vi "SmartLibrary.vi"() -> ()   [LabVIEW 2020]
uses:
  Control 1.ctl
  <vilib>/Utility/file.llb/Read Delimited Spreadsheet (string).vi
panel:
  in  "?":T1(tab)
  out "Misplaced":u8(slide) scale=0.0..100.0
  in  "ENTER BOOK TITLE":string
  out "Current Date and Time":timestamp format="%<%X\n%x>T"
  in  "Search Button":bool
  out "Available":u8(slide) scale=0.0..100.0
  out "Borrowed":u8(slide) scale=0.0..100.0
  in  "RFID 1":bool
  in  "RFID 2":bool
  in  "RFID 3":bool
  in  "RFID 4":bool
  in  "RFID 5":bool
  in  "RFID 6":bool
  in  "RFID 7":bool
  in  "RFID 8":bool
  out "ONLINE":bool
  out "OFFLINE":bool
  out "Author:":string
  out "Call mumber:":string
  out "ISBN/ISSN:":string
  in  "Select\nCSV Database":T2 caption="file path (dialog if empty)"
  # "Book Inventory %"
  # "BOOKS"
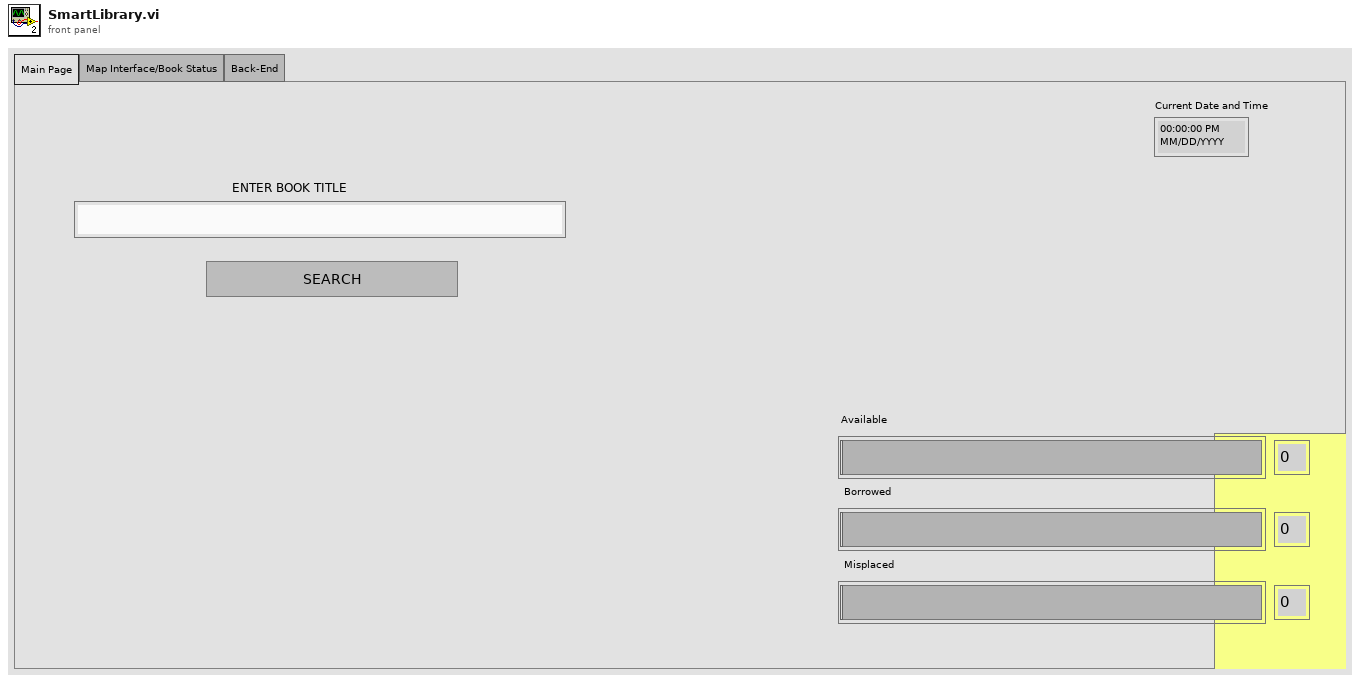
[diagram p1: front panel]
types:
  T1 = enum32{"Main Page", "Map Interface/Book Status", "Back-End"}
  T2 = typedef "Control 1.ctl" = path
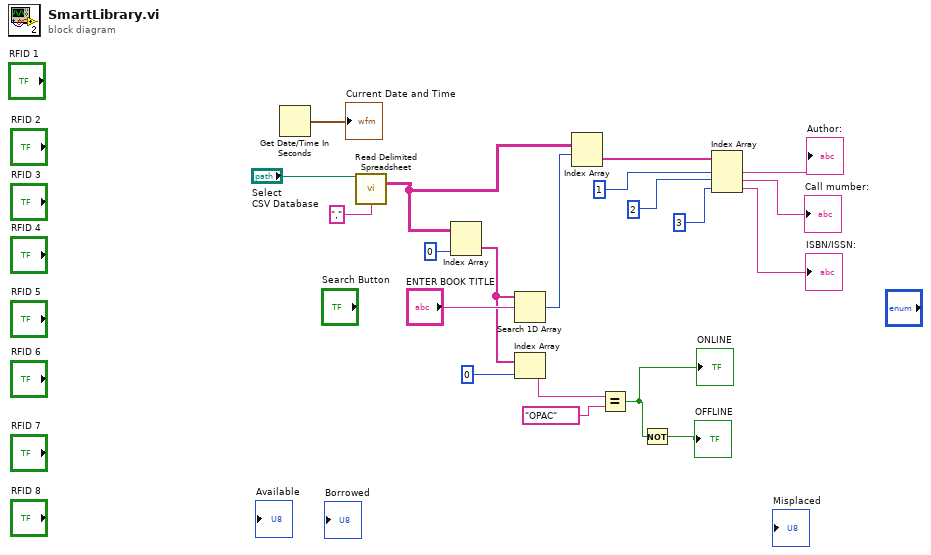
[diagram p0: block diagram]
diagram:
  n1 = Get Date/Time In Seconds() -> (seconds since 1Jan1904=→"Current Date and Time":timestamp)
  n2 = call-poly <vilib>:"Read Delimited Spreadsheet.vi"("file path (dialog if empty)"="Select\nCSV Database", "delimiter (\\t)"="," ("delimiter (\\t)")) -> ("all rows"=w2:string[][])  [unwired: 8 in, 5 out]
  n3 = Index Array(array=w2, index (col)=0 ("disabled index (col)")) -> (element=w7:string[])  [unwired: 1 in]
  n4 = Search 1D Array(1D array=w7, element="ENTER BOOK TITLE") -> (index of element=w18:i32)  [unwired: 1 in]
  n5 = Index Array(array=w7, index=0 ("disabled index (col)")) -> (element=w6:string)
  n6 = Index Array(array=w2, index (row)=w18) -> (element=w17:string[])  [unwired: 1 in]
  n7 = Equal?(x=w6, y="OPAC") -> (x = y?=w3:bool)
  "ONLINE" <- w3
  n8 = Not(x=w3) -> (.not. x?=→"OFFLINE":bool)
  n9 = Index Array(array=w17, index #1=1 ("index"), index #2=2 ("index"), index #3=3 ("index")) -> (element #1=→"Author:":string, element #2=→"Call mumber:":string, element #3=→"ISBN/ISSN:":string)
